vi "模式一.vi"(0 "Input Handle":cluster{"Session":u32, "Card number":u32}, 5 "文件夹路径":path caption="路径", 7 "设置":T1, 11 "error in":errorcluster {"code" format="%.0x"}) -> (4 "Output Handle":cluster{"Session":u32, "Card number":u32}, 15 "error out":errorcluster caption="error in")   [LabVIEW 2018]
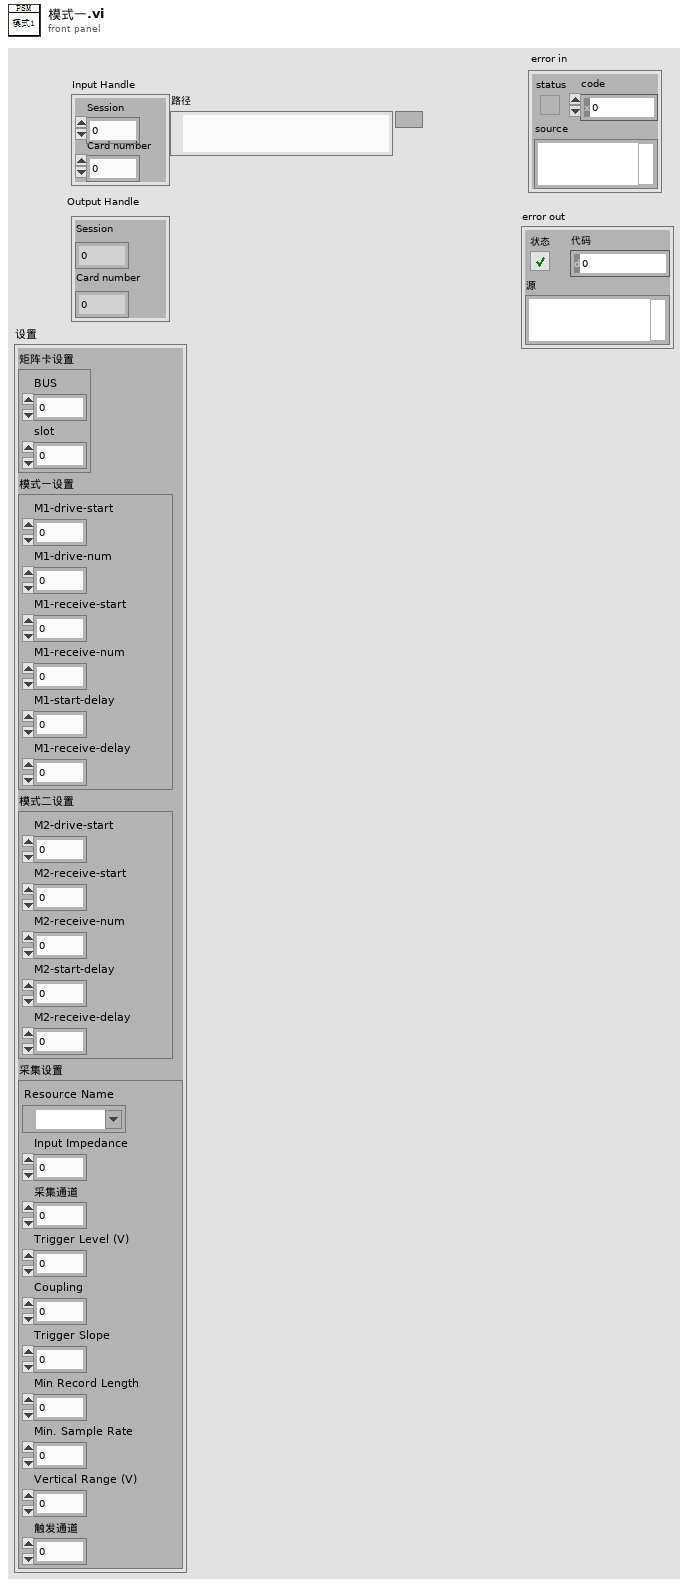
[diagram p1: front panel]
types:
  T1 = cluster{"矩阵卡设置":cluster{"BUS":u32, "slot":u32}, "模式一设置":cluster{"M1-drive-start":u32, "M1-drive-num":u32, "M1-receive-start":u32, "M1-receive-num":u32, "M1-start-delay":u32, "M1-receive-delay":u32}, "模式二设置":cluster{"M2-drive-start":u32, "M2-receive-start":u32, "M2-receive-num":u32, "M2-start-delay":u32, "M2-receive-delay":u32}, "采集设置":cluster{"Resource Name":refnum<k15>, "Input Impedance":u32, "采集通道":i32, "Trigger Level (V)":dbl, "Coupling":u16, "Trigger Slope":i32, "Min Record Length":i32, "Min. Sample Rate":dbl, "Vertical Range (V)":dbl, "触发通道":i32}}
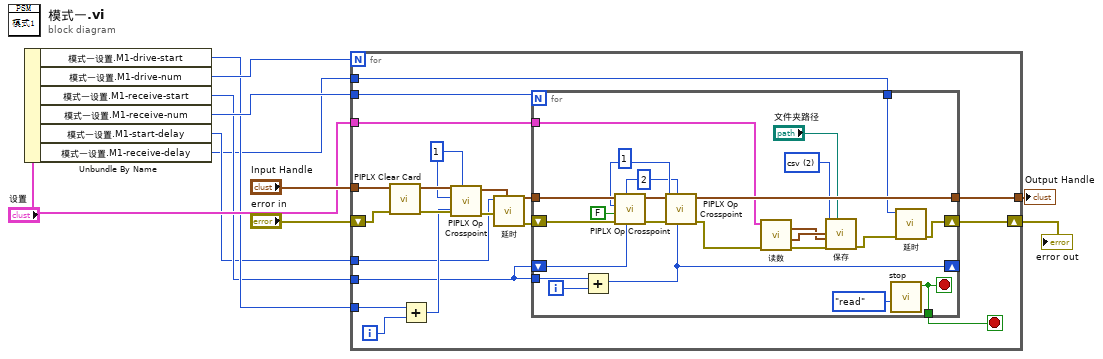
[diagram p0: block diagram]
diagram:
  n1 = Unbundle By Name("设置") -> ("模式一设置.M1-drive-start"=w4:u32, "模式一设置.M1-drive-num"=w6:u32, "模式一设置.M1-receive-start"=w3:u32, "模式一设置.M1-receive-num"=w5:u32, "模式一设置.M1-start-delay"=w2:u32, "模式一设置.M1-receive-delay"=w1:u32)
  n2 = for {
    N: w6 -> [_]
    tunnel: "Input Handle" -> [w28]
    shift-right: [w19] -> w8
    shift-left: "error in" -> [w27]
    tunnel: [w30] -> w9
    tunnel: "设置" -> [w17]
    tunnel: w5 -> [w16]
    tunnel: w4 -> [w15]
    tunnel: w3 -> [w14]
    tunnel: w2 -> [w13]
    tunnel: w1 -> [w12]
    i -> [w20]
    stop <- w29 stop-if-true
    w21 = u32 1 ("Row")
    n3 = call <instrlib>:"PIPLX Clear Card.vi"("error in"=w27, "Input Handle"=w28) -> ("error out"=w26:errorcluster, "Output Handle"=w25:cluster{"Session":u32, "Card number":u32})  [unwired: 8 in]
    n4 = Add(x=w15, y=w20) -> (x+y=w18:u32)
    n5 = call <instrlib>:"PIPLX Op Crosspoint.vi"("Column"=w18, "Row"=w21, "error in"=w26, "Output Subunit"=w21, "Input Handle"=w25) -> ("error out"=w23:errorcluster, "Output Handle"=w24:cluster{"Session":u32, "Card number":u32})  [unwired: 5 in]
    n6 = call "延时.vi"("error in (no error)"=w23, "延时（百毫秒）"=w13) -> ("error out"=w22:errorcluster)  [unwired: 9 in]
    n7 = for {
      N: w16 -> [_]
      tunnel: w24 -> [w54]
      shift-right: [w44] -> w19
      shift-left: w22 -> [w53]
      tunnel: [w50] -> w30
      tunnel: [w52] -> w29
      shift-right: [w46] -> _
      shift-left: w14 -> [w45]
      tunnel: w14 -> [w42]
      tunnel: w17 -> [w33]
      tunnel: w12 -> [w32]
      i -> [w47]
      stop <- w52 stop-if-true
      w38 = u16 2 items=["txt", "xls", "csv", "xlsx"] ("文件类型")
      w40 = u32 2 ("Row")
      w48 = u32 1 ("Output Subunit")
      n8 = Add(x=w42, y=w47) -> (x+y=w46:u32)
      n9 = call <instrlib>:"PIPLX Op Crosspoint.vi"("Column"=w45, "Row"=w40, "error in"=w53, "Action"=FALSE, "Output Subunit"=w48, "Input Handle"=w54) -> ("error out"=w41:errorcluster, "Output Handle"=w49:cluster{"Session":u32, "Card number":u32})  [unwired: 4 in]
      n10 = call <instrlib>:"PIPLX Op Crosspoint.vi"("Column"=w46, "Row"=w40, "error in"=w41, "Output Subunit"=w48, "Input Handle"=w49) -> ("error out"=w39:errorcluster, "Output Handle"=w50:cluster{"Session":u32, "Card number":u32})  [unwired: 5 in]
      n11 = call "读数.vi"("error in"=w39, "设置"=w33) -> ("error out"=w37:errorcluster, "响应信号"=w36:waveform(dbl), "触发信号"=w35:waveform(dbl))  [unwired: 7 in]
      n12 = call "保存.vi"("文件夹路径"="文件夹路径", "error in (no error)"=w37, "激励信号"=w35, "采集信号"=w36, "文件类型"=w38) -> ("error out"=w34:errorcluster)  [unwired: 6 in]
      n13 = call "stop.vi"("枚举"=enum16{"write", "read"}."read") -> ("停止"=w52:bool)  [unwired: 10 in]
      n14 = call "延时.vi"("error in (no error)"=w34, "延时（百毫秒）"=w32) -> ("error out"=w44:errorcluster)  [unwired: 9 in]
    }
  }
  "Output Handle" <- w9
  "error out" <- w8
